vi "Exceltime2LVtime.vi"(3 "ExcelDatetime String":string) -> (0 "LabVIEW Time":timestamp, 1 "date/time string":string)   [LabVIEW 2021]
doc: "transfer excel datetime (number format) to Labview Datetime.\n2015-02-04 11:00:20\n蒋松\njiangsong@outlook.com"
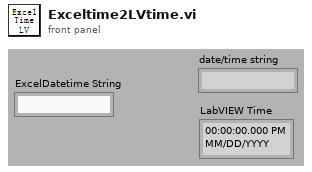
[diagram p1: front panel]
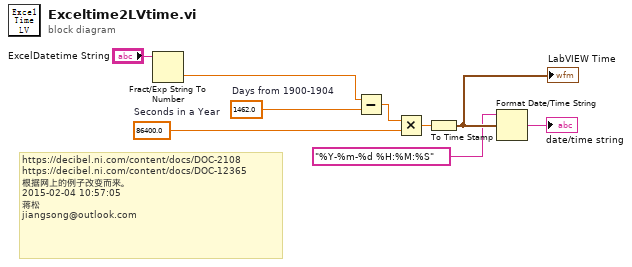
[diagram p0: block diagram]
diagram:
  w9 = 1462.0  # Days from 1900-1904
  w7 = 86400.0  # Seconds in a Year
  # "https://decibel.ni.com/content/docs/DOC-2108\nhttps://decibel.ni.com/content/docs/DOC-12365\n根据网上的例子改变而来。\n2015-02-04 10:57:05\n蒋松\njiangsong@outlook.com"
  n1 = Fract/Exp String To Number(string="ExcelDatetime String") -> (number=w4:dbl)  [unwired: 3 in, 1 out]
  n2 = Subtract(x=w4, y=w9) -> (x-y=w8:dbl)
  n3 = Multiply(x=w8, y=w7) -> (x*y=w6:dbl)
  n4 = To Time Stamp(1:w6) -> (0:w3:timestamp)
  "LabVIEW Time" <- w3
  n5 = Format Date/Time String ("InputDatetime")(time format string (%c)="%Y-%m-%d %H:%M:%S", seconds (now)=w3) -> (date/time string=→"date/time string":string)  [unwired: 1 in]
